vi "Import.vi"(8 "error in (no error)":errorcluster, 11 "BluelinesRedlines in":refnum<class "BluelinesRedlines.lvclass">) -> (0 "error out":errorcluster, 3 "BluelinesRedlines out":refnum<class "BluelinesRedlines.lvclass">)   [LabVIEW 2020, in "VolatusGUIElements.lvlib" / "BluelinesRedlines.lvclass"]
uses:
  BluelinesRedlines.lvclass
  BluelinesRedlines.lvclass/BluelinesRedlines.ctl
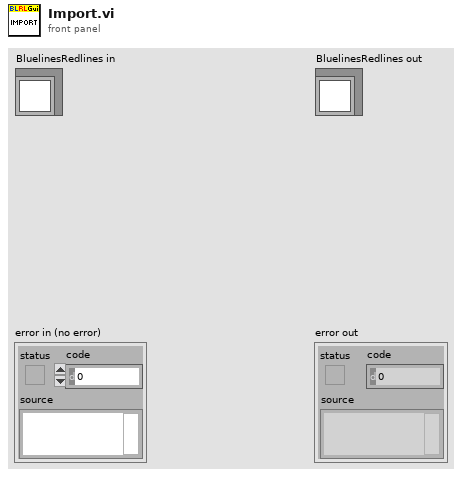
[diagram p1: front panel]
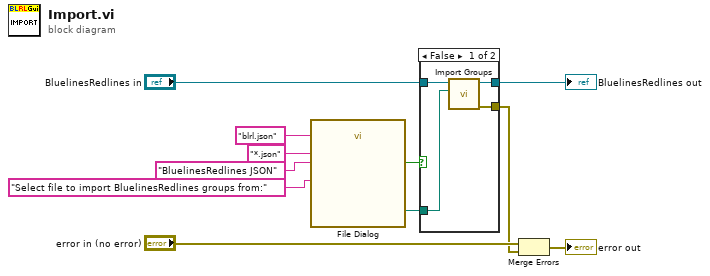
[diagram p0: block diagram]
diagram:
  n1 = call "File Dialog"("prompt"="Select file to import BluelinesRedlines groups from:", "default name"="blrl.json", "pattern (all files)"="*.json", "pattern label"="BluelinesRedlines JSON") -> ("selected path"=w4:path, "cancelled"=w3:bool)  [unwired: 8 in, 2 out]
  n2 = case shown="False" w3 {
    tunnel: "BluelinesRedlines in" -> [w15 w16]
    tunnel: [w14 w16] -> w5
    tunnel: w4 -> [w13 _]
    tunnel: [w12 _] -> w1
    frame False {
      n3 = call "Import Groups.vi"("Path"=w13, "BluelinesRedlines in"=w15) -> ("error out"=w12:errorcluster, "BluelinesRedlines out"=w14:refnum<class "BluelinesRedlines.lvclass">)  [unwired: 8 in]
    }
    frame True {
    }
  }
  "BluelinesRedlines out" <- w5
  n4 = Merge Errors("error in (no error)", w1) -> (→"error out":errorcluster)
